vi "Module Data Acquisition Loop - NLHQ.vi"(7 "Sampling Period (S)":dbl=0.05 caption="采样周期（秒）", 8 "error in (no error)":errorcluster caption="错误输入（无错误）", 11 "Message Queues":T1 caption="消息队列") -> (0 "error out":errorcluster caption="错误输出")   [LabVIEW 2015]
uses:
  Support VIs/Message Queue/All Real-Time Message Queues.ctl
  Support VIs/Message Queue/Message Cluster.ctl
  <vilib>/Platform/TimedLoop/XDataNode/timing_clust.ctl
  <vilib>/Platform/TimedLoop/XDataNode/nitl_modes.ctl
  <vilib>/Platform/TimedLoop/XDataNode/wakeup.ctl
  Globals/Global - Monitoring Variables.vi
  <vilib>/Platform/TimedLoop/XDataNode/loadnilvce.vi
  Globals/Global - All RT Loop Stop.vi
  <vilib>/Platform/TimedLoop/XDataNode/XDataNode.xnode
  <vilib>/Platform/TimedLoop/XDataNode/XDNodeRunTimeDep.lvlib
  Support VIs/Message Queue/Message Queue.lvlib
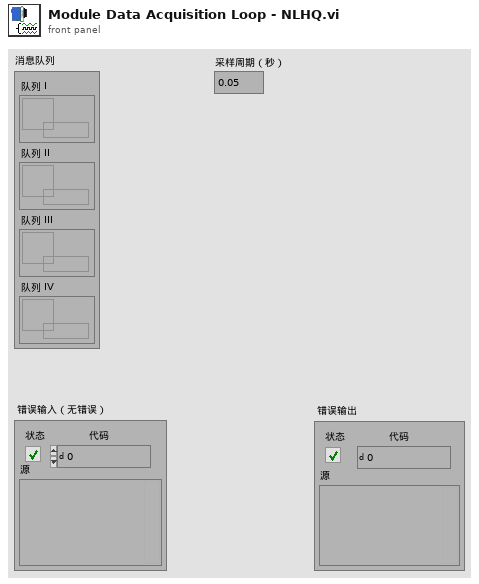
[diagram p1: front panel]
types:
  T1 = typedef "Message Queue.lvlib/All Real-Time Message Queues.ctl" = cluster{"Queue I":refnum<queue>, "Queue II":refnum<queue>, "Queue III":refnum<queue>, "Queue IV":refnum<queue>}
  T2 = typedef "XDNodeRunTimeDep.lvlib/timing_clust.ctl" = cluster{"Expected End [f-1]":u64, "Actual End [f-1]":u64, "Finished Late? [f-1]":bool, "Expected End [i-1]":u64, "Actual End [i-1]":u64, "Finished Late? [i-1]":bool, "Expected Start [i]":u64, "Actual Start [i]":u64, "Expected Start [f]":u64, "Actual Start [f]":u64, "Source Name":string, "Structure Name":string, "Period":i64, "Deadline":i64, "Offset":i64, "Start":i64, "Priority":i32, "Timeout":i32, "Mode":T3, "Wakeup Reason":T4, "Error":errorcluster, "Source Type":string, "Secondary Source Type":string, "Global End Time":u64, "Global Start Time":u64, "Frame Duration":u64, "Iteration Duration":u64, "Assigned CPU":i32, "I/O Scan Engine Mode":u32}
  T3 = typedef "XDNodeRunTimeDep.lvlib/nitl_modes.ctl" = enum32{"No Change", "Process missed periods, maintain original phase", "Discard missed periods, maintain original phase", "Process missed periods, ignore original phase", "Discard missed periods, ignore original phase"}
  T4 = typedef "XDNodeRunTimeDep.lvlib/wakeup.ctl" = enum32{"Normal", "Aborted", "Asynchronous wakeup", "Timing source error", "Timed loop error", "Timeout"}
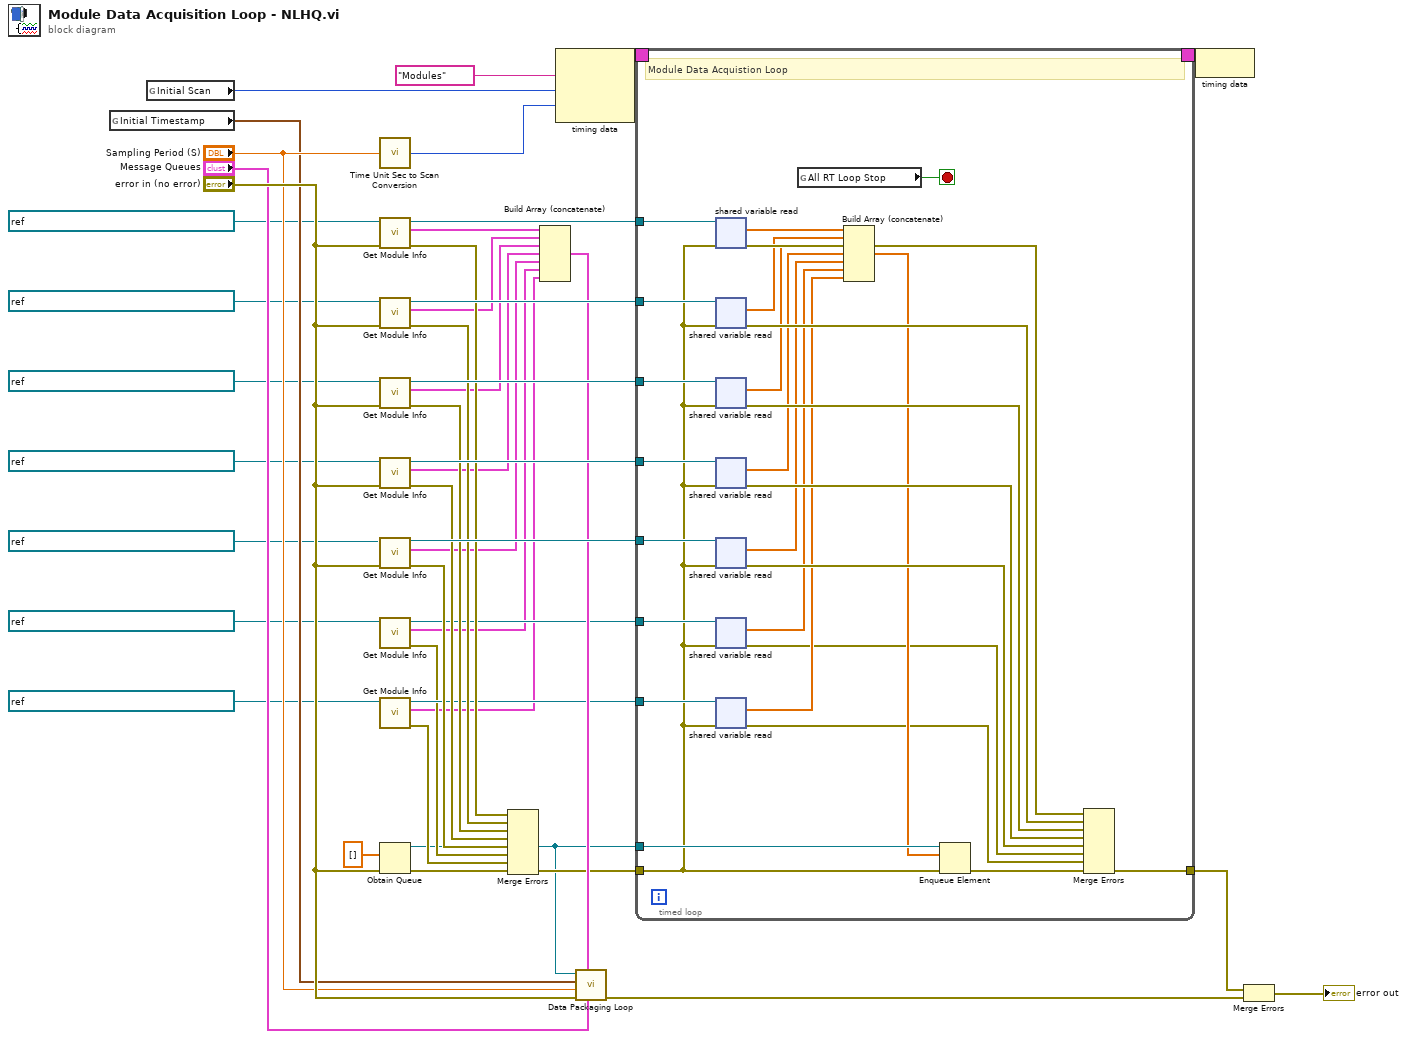
[diagram p0: block diagram]
diagram:
  n1 = global read "Global - Monitoring Variables.vi" "Initial Timestamp"() -> (w21:timestamp)
  n2 = global read "Global - Monitoring Variables.vi" "Initial Scan"() -> (w28:i64)
  n3 = call "Time Unit Sec to Scan Conversion.vi"("time duration (s)"="Sampling Period (S)") -> ("time duration (scan)"=w27:i64)
  n4 = call "Get Module Info.vi"("IO Container"=refnum<k21> "ni.var.io://ni-crio-9036-nlhq/Mod1" ("9239引用句柄"), "error in (no error)"="error in (no error)") -> ("IO Container(dup)"=w40:refnum<k21>, "channel info array"=w35:cluster{"Module":string, "Channel":string}[], "error out"=w34:errorcluster)  [unwired: 6 in]
  n5 = call "Get Module Info.vi"("IO Container"=refnum<k21> "ni.var.io://ni-crio-9036-nlhq/Mod2" ("9219引用句柄"), "error in (no error)"="error in (no error)") -> ("IO Container(dup)"=w39:refnum<k21>, "channel info array"=w4:cluster{"Module":string, "Channel":string}[], "error out"=w33:errorcluster)  [unwired: 6 in]
  n6 = call "Get Module Info.vi"("IO Container"=refnum<k21> "ni.var.io://ni-crio-9036-nlhq/Mod3" ("9219引用句柄"), "error in (no error)"="error in (no error)") -> ("IO Container(dup)"=w38:refnum<k21>, "channel info array"=w5:cluster{"Module":string, "Channel":string}[], "error out"=w32:errorcluster)  [unwired: 6 in]
  n7 = call "Get Module Info.vi"("IO Container"=refnum<k21> "ni.var.io://ni-crio-9036-nlhq/Mod4" ("9219引用句柄"), "error in (no error)"="error in (no error)") -> ("IO Container(dup)"=w37:refnum<k21>, "channel info array"=w6:cluster{"Module":string, "Channel":string}[], "error out"=w31:errorcluster)  [unwired: 6 in]
  n8 = call "Get Module Info.vi"("IO Container"=refnum<k21> "ni.var.io://ni-crio-9036-nlhq/Mod5" ("9219引用句柄"), "error in (no error)"="error in (no error)") -> ("IO Container(dup)"=w36:refnum<k21>, "channel info array"=w7:cluster{"Module":string, "Channel":string}[], "error out"=w30:errorcluster)  [unwired: 6 in]
  n9 = call "Get Module Info.vi"("IO Container"=refnum<k21> "ni.var.io://ni-crio-9036-nlhq/Mod6" ("9219引用句柄")) -> ("IO Container(dup)"=w15:refnum<k21>, "channel info array"=w9:cluster{"Module":string, "Channel":string}[], "error out"=w13:errorcluster)  [unwired: 7 in]
  n10 = call "Get Module Info.vi"("IO Container"=refnum<k21> "ni.var.io://ni-crio-9036-nlhq/Mod7" ("9219引用句柄")) -> ("IO Container(dup)"=w14:refnum<k21>, "channel info array"=w8:cluster{"Module":string, "Channel":string}[], "error out"=w12:errorcluster)  [unwired: 7 in]
  n11 = Obtain Queue(element data type=dbl[] [] ("数据类型"), error in (no error)="error in (no error)") -> (queue out=w3:refnum<queue>, error out=w11:errorcluster)  [unwired: 3 in, 1 out]
  n12 = Merge Errors(w34, w33, w32, w31, w30, w13, w12, w11) -> (w10:errorcluster)
  n13 = Build Array (concatenate)(w35, w4, w5, w6, w7, w9, w8) -> (w25:cluster{"Module":string, "Channel":string}[])
  n14 = node-c288("Modules" ("结构名称"), w28, w27) -> (w45:T2)
  n15 = call "Data Packaging Loop.vi"("Message Queues"="Message Queues", "channel info array"=w25, "error in (no error)"="error in (no error)", "sampling period (s)"="Sampling Period (S)", "timestamp"=w21, "data queue"=w3) -> ("error out"=w26:errorcluster)  [unwired: 5 in]
  n16 = timed-loop {
    timing: w45 -> [_]
    timing-out: [_] -> w44
    tunnel: w3 -> [w71]
    tunnel: [w46] -> w41
    tunnel: w40 -> [w59]
    tunnel: w39 -> [w58]
    tunnel: w38 -> [w57]
    tunnel: w37 -> [w56]
    tunnel: w36 -> [w55]
    tunnel: w10 -> [w52]
    tunnel: w15 -> [w54]
    tunnel: w14 -> [w53]
    stop <- w72 stop-if-true
    # "Module Data Acquistion Loop"
    n17 = shared-variable-read(w59, w52) -> (w66:errorcluster, w65:dbl[])  [unwired: 1 out]
    n18 = shared-variable-read(w58, w52) -> (w67:errorcluster, w64:dbl[])  [unwired: 1 out]
    n19 = shared-variable-read(w57, w52) -> (w68:errorcluster, w63:dbl[])  [unwired: 1 out]
    n20 = shared-variable-read(w56, w52) -> (w69:errorcluster, w62:dbl[])  [unwired: 1 out]
    n21 = shared-variable-read(w55, w52) -> (w70:errorcluster, w61:dbl[])  [unwired: 1 out]
    n22 = shared-variable-read(w54, w52) -> (w49:errorcluster, w51:dbl[])  [unwired: 1 out]
    n23 = shared-variable-read(w53, w52) -> (w48:errorcluster, w50:dbl[])  [unwired: 1 out]
    n24 = global read "Global - All RT Loop Stop.vi" "All RT Loop Stop"() -> (w72:bool)
    n25 = Build Array (concatenate)(w65, w64, w63, w62, w61, w51, w50) -> (w60:dbl[])
    n26 = Enqueue Element(queue=w71, element=w60, error in (no error)=w52) -> (error out=w47:errorcluster)  [unwired: 1 in, 2 out]
    n27 = Merge Errors(w66, w67, w68, w69, w70, w49, w48, w47) -> (w46:errorcluster)
  }
  n28 = node-c288(w44) -> ()
  n29 = Merge Errors(w41, w26) -> (→"error out":errorcluster)
